vi "NumericCommand_Example.vi"() -> ()   [LabVIEW 2019]
uses:
  <vilib>/Rock Robotics/WPI/ThirdParty/JAS_Junk/TrajLib/TypeDef/CHASSIS_SPEEDS.ctl
  <vilib>/Rock Robotics/WPI/ThirdParty/JAS_Junk/TrajLib/VI/numCmd_Recv_Generic.vi
  <vilib>/Rock Robotics/WPI/ThirdParty/JAS_Junk/TrajLib/VI/numCmd_Send_Generic.vi
  <vilib>/Rock Robotics/WPI/ThirdParty/JAS_Junk/TrajLib/VI/numCmd_ObtainQueue.vi
  <vilib>/Rock Robotics/WPI/ThirdParty/JAS_Junk/TrajLib/VI/numCmd_Send_Internal.vi
  <vilib>/Rock Robotics/WPI/ThirdParty/JAS_Junk/TrajLib/Trajectory_Library.lvlib
panel:
  out "Single Value 1\nRead":dbl
  out "Single Value 2\nRead":dbl
  out "Single Value 1\nChanged":bool
  out "Single Value 2\nChanged":bool
  out "Two Values 1\nRead":dbl
  out "Two Values\nChanged":bool
  out "Two Values 2\nRead":dbl
  out "Value Array\nRead":dbl[](array[numeric])
  out "Value Array\nChanged":bool
  out "Chassis Speed\nDemand Changed":bool
  out "Chassis Speed\nDemand Read":T1 {"vOmega" format="%10.3f"; "vY" format="%10.3f"; "vX" format="%10.3f"}
  in  "Single Value 1":dbl
  in  "Single Value 2":dbl
  in  "Two Values 1":dbl
  in  "Two Values 2":dbl
  in  "Value Array":dbl[](array[numeric])
  in  "Chassis Speed \nDemand":T1 {"vOmega" format="%10.3f"; "vY" format="%10.3f"; "vX" format="%10.3f"}
  out "Waveform Chart":cluster{i16, i16, i16, i16, i16}(graph)
  # "NUMERIC COMMAND EXMPLE"
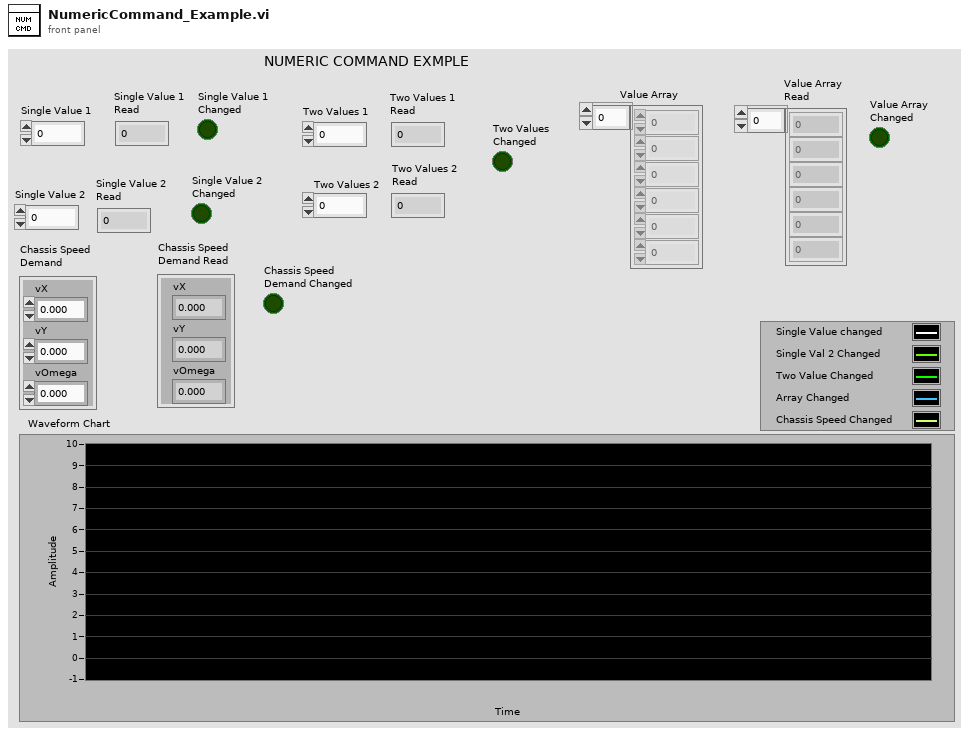
[diagram p1: front panel]
types:
  T1 = typedef "Trajectory_Library.lvlib/CHASSIS_SPEEDS.ctl" = cluster{"vX":dbl, "vY":dbl, "vOmega":dbl}
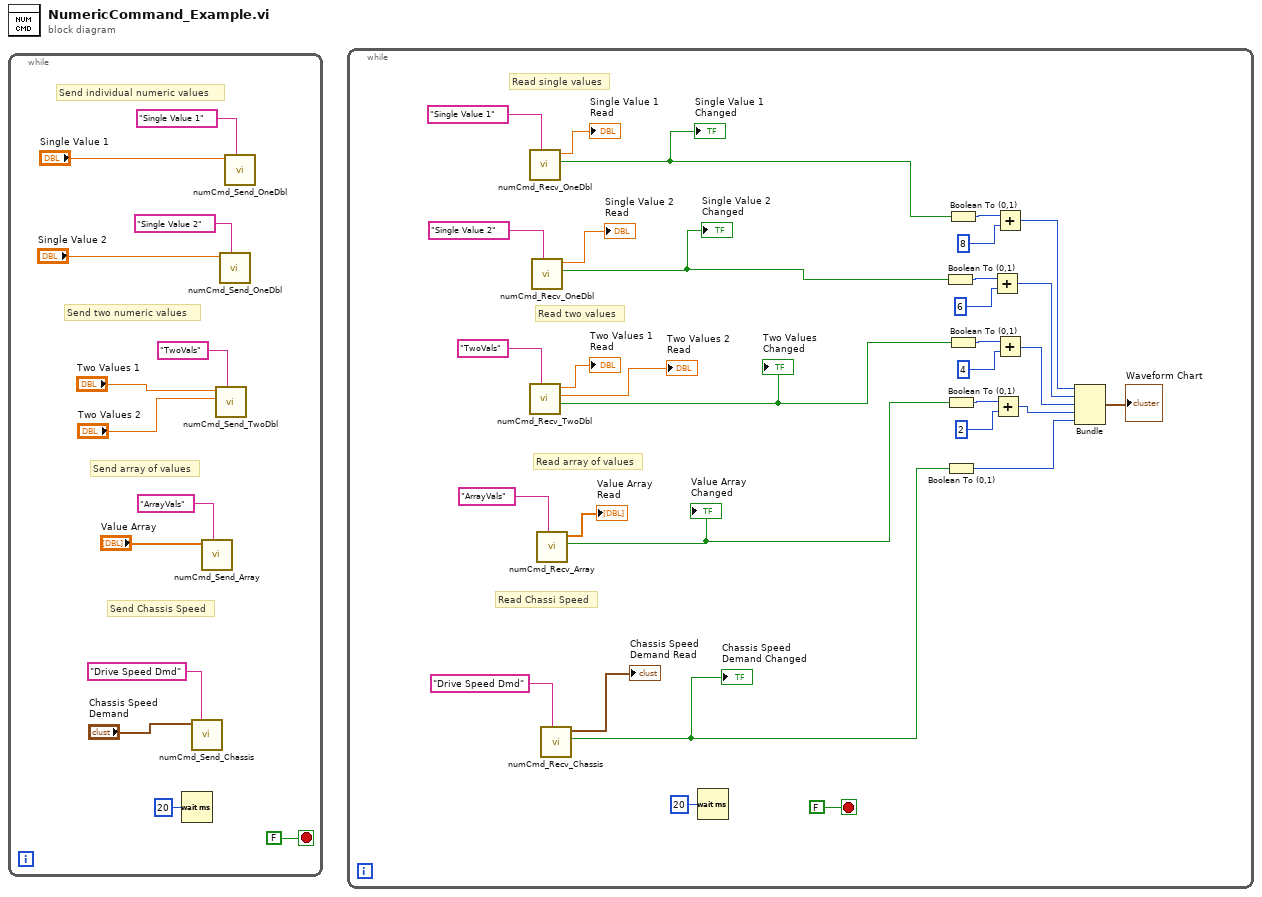
[diagram p0: block diagram]
diagram:
  n1 = while {
    stop <- FALSE stop-if-true
    # "Send Chassis Speed"
    # "Send array of values"
    # "Send two numeric values"
    # "Send individual numeric values"
    n2 = Wait (ms)(milliseconds to wait=u32 20) -> ()  [unwired: 1 out]
    n3 = call <vilib>:"numCmd_Send_Chassis.vi"("Command Name"="Drive Speed Dmd", "Chassis Speeds"="Chassis Speed \nDemand") -> ()  [unwired: 9 in, 1 out]
    n4 = call <vilib>:"numCmd_Send_Array.vi"("Command Name"="ArrayVals", "Values"="Value Array") -> ()  [unwired: 9 in, 1 out]
    n5 = call <vilib>:"numCmd_Send_TwoDbl.vi"("Command Name"="TwoVals", "Value 2"="Two Values 2", "Value 1"="Two Values 1") -> ()  [unwired: 8 in, 1 out]
    n6 = call <vilib>:"numCmd_Send_OneDbl.vi"("Command Name"="Single Value 2", "Value"="Single Value 2") -> ()  [unwired: 9 in, 1 out]
    n7 = call <vilib>:"numCmd_Send_OneDbl.vi"("Command Name"="Single Value 1", "Value"="Single Value 1") -> ()  [unwired: 9 in, 1 out]
  }
  n8 = while {
    stop <- FALSE stop-if-true
    # "Read Chassi Speed"
    # "Read array of values"
    # "Read two values"
    # "Read single values"
    n9 = call <vilib>:"numCmd_Recv_OneDbl.vi"("Command Name"="Single Value 1") -> ("Changed"=w21:bool, "Value"=→"Single Value 1\nRead":dbl)  [unwired: 8 in, 1 out]
    "Single Value 1\nChanged" <- w21
    n10 = call <vilib>:"numCmd_Recv_TwoDbl.vi"("Command Name"="TwoVals") -> ("Any Changed"=w19:bool, "Value 2"=→"Two Values 2\nRead":dbl, "Value 1"=→"Two Values 1\nRead":dbl)  [unwired: 7 in, 1 out]
    "Two Values\nChanged" <- w19
    n11 = call <vilib>:"numCmd_Recv_OneDbl.vi"("Command Name"="Single Value 2") -> ("Changed"=w20:bool, "Value"=→"Single Value 2\nRead":dbl)  [unwired: 8 in, 1 out]
    "Single Value 2\nChanged" <- w20
    n12 = call <vilib>:"numCmd_Recv_Array.vi"("Command Name"="ArrayVals") -> ("Any Changed"=w18:bool, "Values"=→"Value Array\nRead":dbl[])  [unwired: 8 in, 1 out]
    "Value Array\nChanged" <- w18
    n13 = call <vilib>:"numCmd_Recv_Chassis.vi"("Command Name"="Drive Speed Dmd") -> ("Any Changed"=w17:bool, "Chassis Speeds"=→"Chassis Speed\nDemand Read":T1)  [unwired: 8 in, 1 out]
    "Chassis Speed\nDemand Changed" <- w17
    n14 = Wait (ms)(milliseconds to wait=u32 20) -> ()  [unwired: 1 out]
    n15 = Boolean To (0,1)(Boolean=w20) -> (0, 1=w25:i16)
    n16 = Boolean To (0,1)(Boolean=w18) -> (0, 1=w31:i16)
    n17 = Boolean To (0,1)(Boolean=w17) -> (0, 1=w29:i16)
    n18 = Boolean To (0,1)(Boolean=w21) -> (0, 1=w23:i16)
    n19 = Boolean To (0,1)(Boolean=w19) -> (0, 1=w27:i16)
    n20 = Add(x=w25, y=i16 6) -> (x+y=w15:i16)
    n21 = Add(x=w31, y=i16 2) -> (x+y=w30:i16)
    n22 = Add(x=w23, y=i16 8) -> (x+y=w14:i16)
    n23 = Add(x=w27, y=i16 4) -> (x+y=w16:i16)
    n24 = Bundle(w14, w15, w16, w30, w29) -> (→"Waveform Chart":cluster{i16, i16, i16, i16, i16})  [unwired: 1 in]
  }
